vi "Hardware In - Engine State.vi"(5 "Set Safe State":bool, 7 "CrankRanThreshold":sgl, 11 "EPTxData":T1) -> (3 "Engine Status":T2)   [LabVIEW 2015, in "ECS-RT.lvlib"]
uses:
  ECS-RT.lvlib
  Typedefs/EPT/Engine Status.ctl
  <vilib>/Powertrain Controls/Device Drivers/Engine Position Tracking/EPTx/RevA/RT/Controls/EPTxData.ctl
  ECS-Shared.lvlib
  <vilib>/Powertrain Controls/Device Drivers/Engine Position Tracking/EPTx/RevA/RT/EPTx - RevA - RT.lvlib
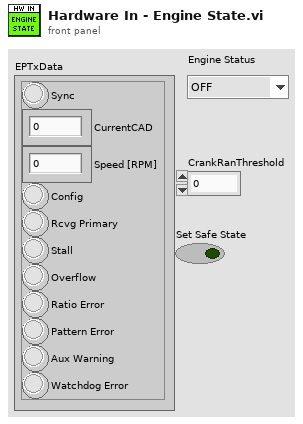
[diagram p1: front panel]
types:
  T1 = typedef "EPTx - RevA - RT.lvlib/EPTxData.ctl" = cluster{"Sync":bool, "CurrentCAD":sgl, "Speed [RPM]":sgl, "Config":bool, "Rcvg Primary":bool, "Stall":bool, "Overflow":bool, "Ratio Error":bool, "Pattern Error":bool, "Aux Warning":bool, "Watchdog Error":bool}
  T2 = typedef "ECS-Shared.lvlib/Engine Status.ctl" = enum16{"OFF", "STALLED", "CRANKING", "RUNNING", "ACCEL", "DECEL", "SAFE"}
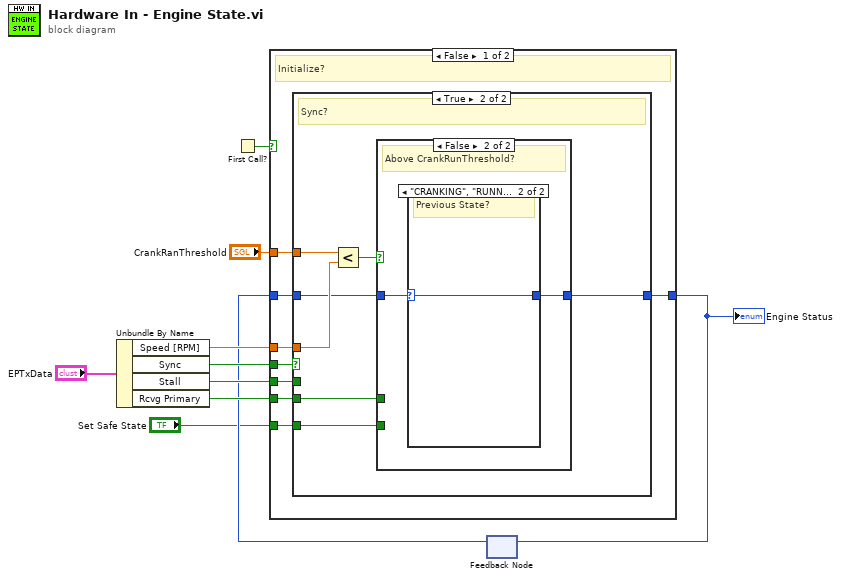
[diagram p0: block diagram]
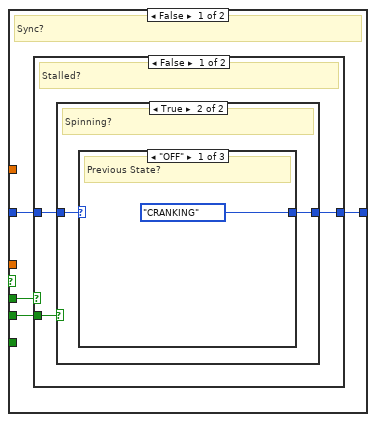
[diagram p2: hidden frame]
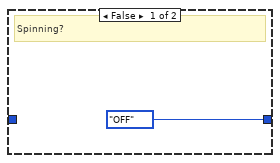
[diagram p3: hidden frame]
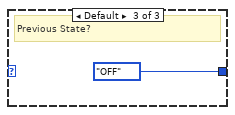
[diagram p5: hidden frame]
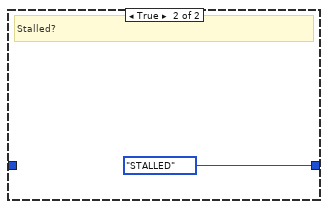
[diagram p6: hidden frame]
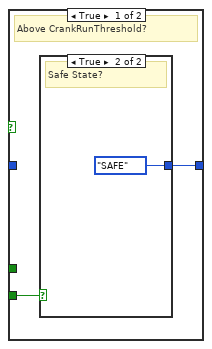
[diagram p7: hidden frame]
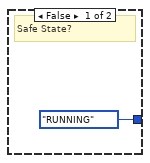
[diagram p8: hidden frame]
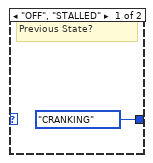
[diagram p9: hidden frame]
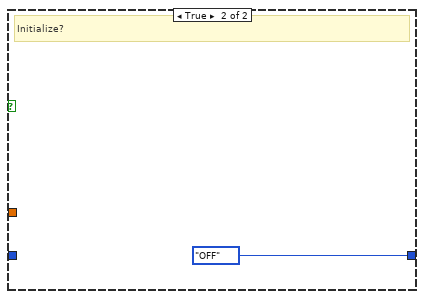
[diagram p10: hidden frame]
diagram:
  n1 = Unbundle By Name("EPTxData") -> ("Speed [RPM]"=w8:sgl, "Sync"=w6:bool, "Stall"=w7:bool, "Rcvg Primary"=w9:bool)
  n2 = First Call?() -> (First Call?: T/F=w10:bool)
  n3 = feedback #1() -> (w4:T2)  [unwired: 1 in]
  n4 = case shown="False" w10 {
    tunnel: w4 -> [w15 _]
    tunnel: [w17 Engine_Status."OFF" ("Engine Status")] -> w5
    tunnel: w7 -> [w18 _]
    tunnel: w6 -> [w14 _]
    tunnel: w9 -> [w16 _]
    tunnel: w8 -> [w13 _]
    tunnel: "Set Safe State" -> [w12 _]
    tunnel: "CrankRanThreshold" -> [w11 _]
    frame False {
      # "Initialize?"
      n5 = case shown="True" w14 {
        tunnel: w18 -> [w21 _]
        tunnel: [w22 w39] -> w17
        tunnel: w16 -> [w20 w38]
        tunnel: w15 -> [w19 w33]
        tunnel: w13 -> [_ w35]
        tunnel: w12 -> [_ w37]
        tunnel: w11 -> [_ w34]
        frame False {
          # "Sync?"
          n6 = case shown="False" w21 {
            tunnel: [w23 Engine_Status."STALLED" ("Engine Status")] -> w22
            tunnel: w20 -> [w25 _]
            tunnel: w19 -> [w24 _]
            frame False {
              # "Stalled?"
              n7 = case shown="True" w25 {
                tunnel: [Engine_Status."OFF" ("Engine Status") w27] -> w23
                tunnel: w24 -> [_ w28]
                frame False {
                  # "Spinning?"
                }
                frame True {
                  # "Spinning?"
                  n8 = case shown="\"OFF\"" w28 {
                    selector: w28 -> [_ w30 _]
                    tunnel: [Engine_Status."CRANKING" ("Engine Status") w30 Engine_Status."OFF" ("Engine Status")] -> w27
                    frame "OFF" {
                      # "Previous State?"
                    }
                    frame "CRANKING" {
                      # "Previous State?"
                    }
                    frame Default {
                      # "Previous State?"
                    }
                  }
                }
              }
            }
            frame True {
              # "Stalled?"
            }
          }
        }
        frame True {
          # "Sync?"
          n9 = Less?(x=w34, y=w35) -> (x < y?=w36:bool)
          n10 = case shown="False" w36 {
            tunnel: [w41 w45] -> w39
            tunnel: w38 -> [_ _]
            tunnel: w37 -> [w40 _]
            tunnel: w33 -> [_ w44]
            frame True {
              # "Above CrankRunThreshold?"
              n11 = case shown="True" w40 {
                tunnel: [Engine_Status."RUNNING" ("Engine Status") Engine_Status."SAFE" ("Engine Status")] -> w41
                frame False {
                  # "Safe State?"
                }
                frame True {
                  # "Safe State?"
                }
              }
            }
            frame False {
              # "Above CrankRunThreshold?"
              n12 = case shown="\"CRANKING\", \"RUNNING\", Default" w44 {
                selector: w44 -> [_ w47]
                tunnel: [Engine_Status."CRANKING" ("Engine Status") w47] -> w45
                frame "OFF", "STALLED" {
                  # "Previous State?"
                }
                frame "CRANKING", "RUNNING", Default {
                  # "Previous State?"
                }
              }
            }
          }
        }
      }
    }
    frame True {
      # "Initialize?"
    }
  }
  "Engine Status" <- w5
  n13 = feedback-in #1(w5) -> ()
